vi "MagOne_RTref.vi"() -> ()   [LabVIEW 2015]
uses:
  \\ds.leeds.ac.uk\student/student2/mn11dpj/Documents/PhD/Designs/Soft Grasper/MagOne_with_2D scanning/MagOne_with_2D scanning/Controls/Host_I2CBus_Options.ctl
  <vilib>/Platform/TimedLoop/XDataNode/timing_clust.ctl
  <vilib>/Platform/TimedLoop/XDataNode/nitl_modes.ctl
  <vilib>/Platform/TimedLoop/XDataNode/wakeup.ctl
  \\ds.leeds.ac.uk\student/student2/mn11dpj/Documents/PhD/Designs/Soft Grasper/MagOne_with_2D scanning/MagOne_with_2D scanning/FPGA/Controls/i2c_state.ctl
  <vilib>/Platform/TimedLoop/scheduler/LVUserAPI/_suppVIs/Create_1MHz_TSource.vi
  <vilib>/platform/TimedLoop/XDataNode/XDataNode.xnode
  <vilib>/Platform/TimedLoop/XDataNode/XDNodeRunTimeDep.lvlib
panel:
  out "Actual Frequency":dbl
  out "Data Read Graph":cluster{dbl, dbl, dbl}(graph)
  out "Loop Time (us)":u32
  out "Data Read":cluster{"Bx":dbl, "By":dbl, "Bz":dbl}
  out "Reading Status":u8 format="%08b"
  in  "Stop":bool
  in  "Frequency (Hz)":dbl=200.0 min=1.0 max=700.0 step=1.0
  in  "Gain_SEL":T1(ring)=enum."G-3"
  # "Different Gain means different resolution and measuring range\nThe higher the Gain, the higher the resolution, the smaller the measuring range"
  # "XY axis magnetic field:  \nGain=0  Mearuign range: -26.4~+26.4mT   (-264~+264 Gauss)\nGain=3  Mearuign range: -13.2~+13.2mT   (-132~+132 Gauss)\nGain=5  Mearuign range: -8.8~+8.8mT       (-88~+88 Gauss)\nGain=7  Mearuign range: -5.3mT~+5.3mT  (-53~+53 Gauss)"
  # "Z axis magnetic field:  \nGain=0  Mearuign range: -96.2~+96.2mT       (-962~+962 Gauss)\nGain=3  Mearuign range: -48.1~+48.1mT       (-481~+481 Gauss)\nGain=5  Mearuign range: -32.1~+32.1mT       (-321~+321 Gauss)\nGain=7  Mearuign range: -19.2mT~+19.2mT  (-192~+192 Gauss)"
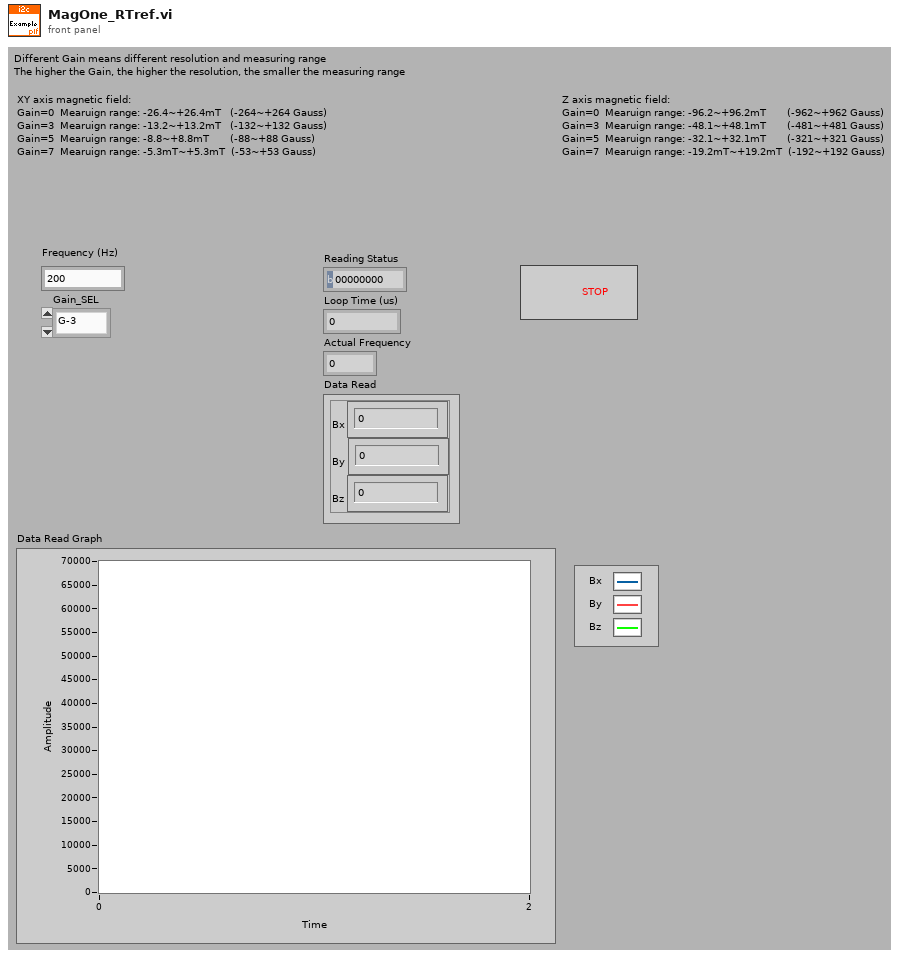
[diagram p1: front panel]
types:
  T1 = enum16{"G-0", "G-1", "G-2", "G-3", "G-4", "G-5", "G-6", "G-7"}
  T2 = typedef "Host_I2CBus_Options.ctl" = enum16{"Open I2C Bus", "Send CMD", "Close I2C Bus"}
  T3 = typedef "i2c_state.ctl" = enum16{"Monitor", "W_To_Device", "R_From_Device", "W/R_From_Device", "TerminateCore"}
  T4 = cluster{"Use_10-Bit_Address":bool, "Slave Device Address":u8, "10-Bit_Address":u8, "NumBytesToRead":i32, "i2c Core Option":T3}
  T5 = typedef "XDNodeRunTimeDep.lvlib/timing_clust.ctl" = cluster{"Expected End [f-1]":u64, "Actual End [f-1]":u64, "Finished Late? [f-1]":bool, "Expected End [i-1]":u64, "Actual End [i-1]":u64, "Finished Late? [i-1]":bool, "Expected Start [i]":u64, "Actual Start [i]":u64, "Expected Start [f]":u64, "Actual Start [f]":u64, "Source Name":string, "Structure Name":string, "Period":i64, "Deadline":i64, "Offset":i64, "Start":i64, "Priority":i32, "Timeout":i32, "Mode":T6, "Wakeup Reason":T7, "Error":errorcluster, "Source Type":string, "Secondary Source Type":string, "Global End Time":u64, "Global Start Time":u64, "Frame Duration":u64, "Iteration Duration":u64, "Assigned CPU":i32, "I/O Scan Engine Mode":u32}
  T6 = typedef "XDNodeRunTimeDep.lvlib/nitl_modes.ctl" = enum32{"No Change", "Process missed periods, maintain original phase", "Discard missed periods, maintain original phase", "Process missed periods, ignore original phase", "Discard missed periods, ignore original phase"}
  T7 = typedef "XDNodeRunTimeDep.lvlib/wakeup.ctl" = enum32{"Normal", "Aborted", "Asynchronous wakeup", "Timing source error", "Timed loop error", "Timeout"}
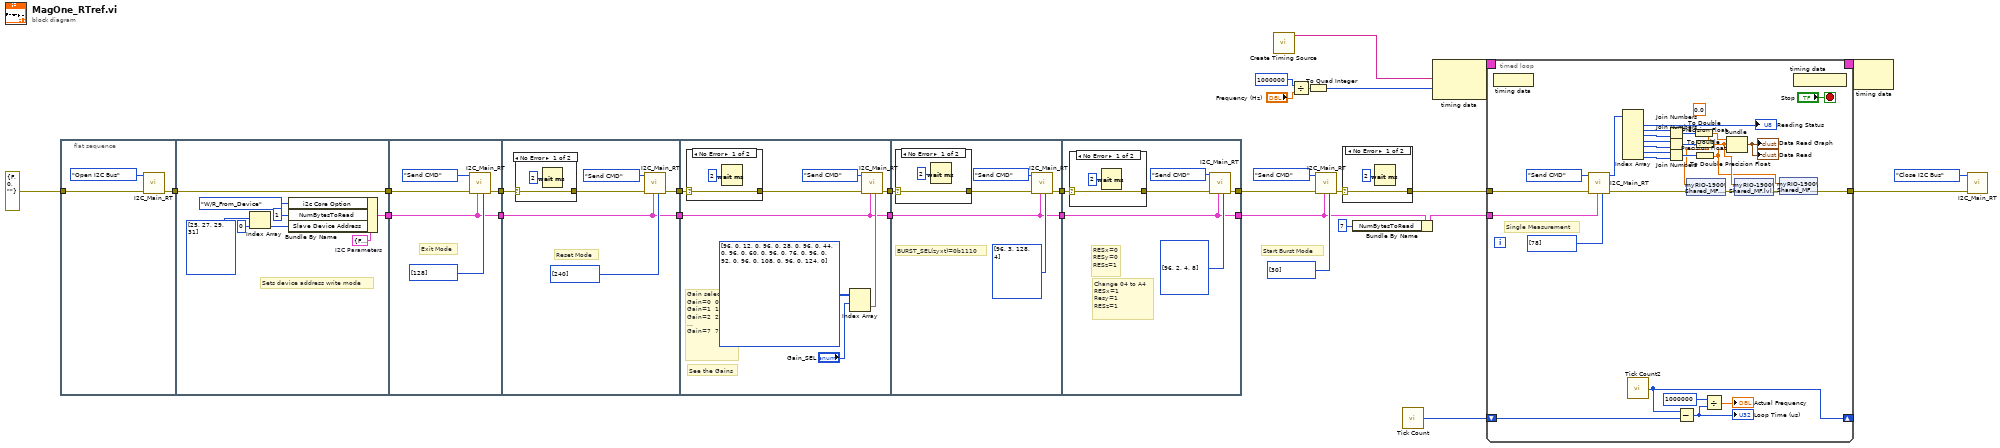
[diagram p0: block diagram]
diagram:
  # "Start Burst Mode"
  n1 = flat-sequence {
    tunnel: [w32] -> w27
    tunnel: errorcluster {"status"=FALSE, "code"=0, "source"=""} ("error constant") -> [w31]
    tunnel: [w41] -> w26
    tunnel: w27 -> [w41]
    tunnel: [w34] -> w7
    tunnel: [w43] -> w25
    tunnel: [w42] -> w24
    tunnel: w26 -> [w45]
    tunnel: w7 -> [w42]
    tunnel: w25 -> [w52]
    tunnel: w24 -> [w47]
    tunnel: [w48] -> w23
    tunnel: [w47] -> w22
    tunnel: w23 -> [w61]
    tunnel: w22 -> [w57]
    tunnel: [w58] -> w21
    tunnel: [w57] -> w20
    tunnel: w21 -> [w70]
    tunnel: w20 -> [w67]
    tunnel: [w68] -> w19
    tunnel: [w67] -> w18
    tunnel: w19 -> [w79]
    tunnel: w18 -> [w76]
    tunnel: [w77] -> w11
    tunnel: [w76] -> w6
    frame #0 {
      n2 = call "I2C_Main_RT.vi"("error in (no error)"=w31, "I2C Bus"=Host_I2CBus_Options."Open I2C Bus") -> ("error out"=w32:errorcluster)  [unwired: 3 in, 6 out]
    }
    frame #1 {
      w37 = T4 {"Use_10-Bit_Address"=FALSE, "Slave Device Address"=160, "10-Bit_Address"=0, "NumBytesToRead"=0, "i2c Core Option"=enum."W_To_Device"}  # I2C Parameters
      # "Sets device address write mode"
      n3 = Index Array(array=u8[] [25, 27, 29, 31] ("CMD_Bytes"), index=0) -> (element=w40:u8)
      n4 = Bundle By Name(cluster=w37, "i2c Core Option"=i2c_state."W/R_From_Device", "NumBytesToRead"=1, "Slave Device Address"=w40) -> (w34:T4)
    }
    frame #2 {
      # "Exit Mode"
      n5 = call "I2C_Main_RT.vi"("CMD_Bytes"=u8[] [128], "I2C Parameters"=w42, "error in (no error)"=w45, "I2C Bus"=Host_I2CBus_Options."Send CMD") -> ("error out"=w43:errorcluster)  [unwired: 1 in, 6 out]
    }
    frame #3 {
      # "Reset Mode"
      n6 = case shown="No Error" w52 {
        selector: w52 -> [w54 w55]
        tunnel: [w54 w55] -> w50
        frame No Error {
          n7 = Wait (ms)(milliseconds to wait=u32 2) -> ()  [unwired: 1 out]
        }
        frame Error {
        }
      }
      n8 = call "I2C_Main_RT.vi"("CMD_Bytes"=u8[] [240], "I2C Parameters"=w47, "error in (no error)"=w50, "I2C Bus"=Host_I2CBus_Options."Send CMD") -> ("error out"=w48:errorcluster)  [unwired: 1 in, 6 out]
    }
    frame #4 {
      # "See the Gains"
      # "Gain selection\nGain=0  0C\nGain=1  1C\nGain=2  2C\n...\nGain=7  7C"
      n9 = case shown="No Error" w61 {
        selector: w61 -> [w65 w66]
        tunnel: [w65 w66] -> w62
        frame No Error {
          n10 = Wait (ms)(milliseconds to wait=u32 2) -> ()  [unwired: 1 out]
        }
        frame Error {
        }
      }
      n11 = Index Array(array=u8[][] [[96, 0, 12, 0], [96, 0, 28, 0], [96, 0, 44, 0], [96, 0, 60, 0], [96, 0, 76, 0], [96, 0, 92, 0], [96, 0, 108, 0], [96, 0, 124, 0]] ("CMD_Bytes"), index (row)="Gain_SEL") -> (element=w59:u8[])  [unwired: 1 in]
      n12 = call "I2C_Main_RT.vi"("CMD_Bytes"=w59, "I2C Parameters"=w57, "error in (no error)"=w62, "I2C Bus"=Host_I2CBus_Options."Send CMD") -> ("error out"=w58:errorcluster)  [unwired: 1 in, 6 out]
    }
    frame #5 {
      # "BURST_SEL(zyxt)=0b1110"
      n13 = case shown="No Error" w70 {
        selector: w70 -> [w74 w75]
        tunnel: [w74 w75] -> w72
        frame No Error {
          n14 = Wait (ms)(milliseconds to wait=u32 2) -> ()  [unwired: 1 out]
        }
        frame Error {
        }
      }
      n15 = call "I2C_Main_RT.vi"("CMD_Bytes"=u8[] [96, 3, 128, 4], "I2C Parameters"=w67, "error in (no error)"=w72, "I2C Bus"=Host_I2CBus_Options."Send CMD") -> ("error out"=w68:errorcluster)  [unwired: 1 in, 6 out]
    }
    frame #6 {
      # "Change 04 to A4\nRESx=1\nResy=1\nRESz=1"
      # "RESx=0\nRESy=0\nRESz=1"
      n16 = case shown="No Error" w79 {
        selector: w79 -> [w83 w84]
        tunnel: [w83 w84] -> w80
        frame No Error {
          n17 = Wait (ms)(milliseconds to wait=u32 2) -> ()  [unwired: 1 out]
        }
        frame Error {
        }
      }
      n18 = call "I2C_Main_RT.vi"("CMD_Bytes"=u8[] [96, 2, 4, 8], "I2C Parameters"=w76, "error in (no error)"=w80, "I2C Bus"=Host_I2CBus_Options."Send CMD") -> ("error out"=w77:errorcluster)  [unwired: 1 in, 6 out]
    }
  }
  n19 = call-poly <vilib>:"Create Timing Source.vi"() -> ("name (out)"=w3:string)  [unwired: 10 in, 1 out]
  n20 = Divide(x=1000000, y="Frequency (Hz)") -> (x/y=w15:dbl)
  n21 = To Quad Integer(1:w15) -> (0:w14:i64)
  n22 = call "I2C_Main_RT.vi"("CMD_Bytes"=u8[] [30], "I2C Parameters"=w6, "error in (no error)"=w11, "I2C Bus"=Host_I2CBus_Options."Send CMD") -> ("error out"=w10:errorcluster)  [unwired: 1 in, 6 out]
  n23 = case shown="No Error" w10 {
    selector: w10 -> [w86 w87]
    tunnel: [w86 w87] -> w9
    frame No Error {
      n24 = Wait (ms)(milliseconds to wait=u32 2) -> ()  [unwired: 1 out]
    }
    frame Error {
    }
  }
  n25 = Bundle By Name(cluster=w6, "NumBytesToRead"=7) -> (w2:T4)
  n26 = call "Tick Count"() -> ("Tick Count(uSec)"=w5:u32)
  n27 = node-c288(w3, w14) -> (w29:T5)
  n28 = timed-loop {
    timing: w29 -> [_]
    timing-out: [_] -> w28
    tunnel: [w91] -> w30
    shift-right: [w99] -> _
    shift-left: w5 -> [w104]
    tunnel: w9 -> [w102]
    tunnel: w2 -> [w100]
    stop <- "Stop" stop-if-true
    (unwired) 0.0
    # "Single Measurement"
    n29 = node-c288 ("Output Node")() -> ()  [unwired: 1 in]
    n30 = call "I2C_Main_RT.vi"("CMD_Bytes"=u8[] [78], "I2C Parameters"=w100, "error in (no error)"=w102, "I2C Bus"=Host_I2CBus_Options."Send CMD") -> ("error out"=w94:errorcluster, "DataBytes"=w114:u8[])  [unwired: 1 in, 5 out]
    n31 = Index Array(array=w114) -> (element #1=→"Reading Status":u8, element #2=w112:u8, element #3=w111:u8, element #4=w110:u8, element #5=w109:u8, element #6=w108:u8, element #7=w107:u8)  [unwired: 7 in]
    n32 = call "Tick Count2"() -> ("Tick Count(uSec)"=w99:u32)
    n33 = Join Numbers(hi=w112, lo=w111) -> ((hi.lo)=w101:u16)
    n34 = Join Numbers(hi=w110, lo=w109) -> ((hi.lo)=w106:u16)
    n35 = Join Numbers(hi=w108, lo=w107) -> ((hi.lo)=w105:u16)
    n36 = Subtract(x=w99, y=w104) -> (x-y=w98:u32)
    "Loop Time (us)" <- w98
    n37 = To Double Precision Float(number=w101) -> (double precision float=w88:dbl)
    n38 = shared-variable "myRIO-1900\\Shared_MF.lvlib\\Bx"(w88, error in=w94) -> (error out=w93:errorcluster)
    n39 = To Double Precision Float(number=w106) -> (double precision float=w90:dbl)
    n40 = To Double Precision Float(number=w105) -> (double precision float=w89:dbl)
    n41 = Divide(x=u32 1000000, y=w98) -> (x/y=→"Actual Frequency":dbl)
    n42 = Bundle(w88, w90, w89) -> (→"Data Read" →"Data Read Graph":cluster{dbl, dbl, dbl})  [unwired: 1 in]
    n43 = shared-variable "myRIO-1900\\Shared_MF.lvlib\\By"(w90, error in=w93) -> (error out=w92:errorcluster)
    n44 = shared-variable "myRIO-1900\\Shared_MF.lvlib\\Bz"(w89, error in=w92) -> (error out=w91:errorcluster)
    n45 = node-c288() -> ()  [unwired: 1 out]
  }
  n46 = node-c288(w28) -> ()  [unwired: 1 out]
  n47 = call "I2C_Main_RT.vi"("error in (no error)"=w30, "I2C Bus"=Host_I2CBus_Options."Close I2C Bus") -> ()  [unwired: 3 in, 7 out]
